vi "SAC-Configure Hardware (TDT).vi"(0 "Params":T1={"Fs (Hz)"=0.0, "atten (dB)"=0.0, "Waveform"=enum."Chirp", "Freq Res (Hz)"=0.0, "Order"=0, "Averages"=0, "seed"=-1, "Window"={"Type"=enum."None", "Length (ms)"=0.0, "Center (ms)"=0.0}, "Mic gain"=0.0, "Mic sens"=0.0}, 11 "error in (no error)":errorcluster) -> (4 "Stimulus":dbl[](array[numeric]), 6 "Sample Rate (Hz)":dbl, 8 "pts/rep":i32, 10 "reps/frame":i32, 15 "error out":errorcluster)   [LabVIEW 2020]
uses:
  Typedefs/SAC-Parameters.ctl
  HRTF VIs/Typedefs/HRTF-Waveform.ctl
  HRTF VIs/Typedefs/HRTF-Window.ctl
  HRTF VIs/Typedefs/HRTF-Window Type.ctl
  PXI DAQ VIs/TDT VIs/TDT-Signal Bank Action.ctl
  Typedefs/SAC-Hardware Config (TDT).ctl
  PXI DAQ VIs/TDT VIs/Typedefs/TDT-Output source.ctl
  PXI DAQ VIs/TDT VIs/Typedefs/TDT-Device ID.ctl
  PXI DAQ VIs/TDT VIs/Typedefs/TDT-Device Config.ctl
  PXI DAQ VIs/TDT VIs/Typedefs/TDT-Input source.ctl
  Utility VIs/Math VIs/dB to Linear (scalar).vi
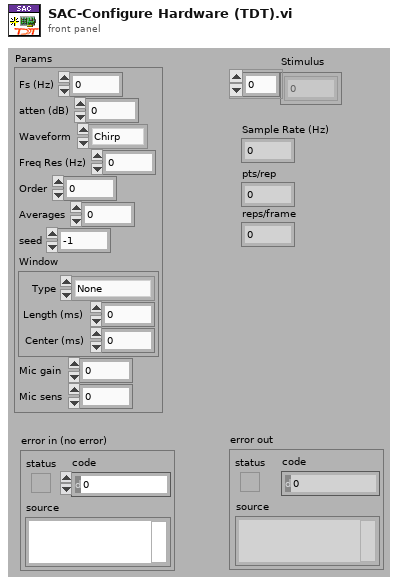
[diagram p1: front panel]
types:
  T1 = typedef "SAC-Parameters.ctl" = cluster{"Fs (Hz)":dbl, "atten (dB)":dbl, "Waveform":T2, "Freq Res (Hz)":dbl, "Order":i32, "Averages":i32, "seed":i64, "Window":T3, "Mic gain":dbl, "Mic sens":dbl}
  T2 = typedef "HRTF-Waveform.ctl" = enum16{"Chirp", "MLS"}
  T3 = typedef "HRTF-Window.ctl" = cluster{"Type":T4, "Length (ms)":dbl, "Center (ms)":dbl}
  T4 = typedef "HRTF-Window Type.ctl" = enum16{"None", "Rectangle", "Hanning"}
  T5 = typedef "TDT-Device Config.ctl" = cluster{"Output":T6, "Input":T8}
  T6 = typedef "TDT-Output source.ctl" = cluster{"Device":T7, "Num":i32}
  T7 = typedef "TDT-Device ID.ctl" = enum16{"None", "PA5", "RP2", "RL2", "RA16", "RV8", "RX5", "RX6", "RX7", "RX8", "RZ2", "RZ5", "RZ6"}
  T8 = typedef "TDT-Input source.ctl" = enum16{"Front Panel", "RA4LI", "RA16LI"}
  T9 = typedef "SAC-Hardware Config (TDT).ctl" = cluster{"Output":T6, "Speaker":cluster{"Channel":i32, "Primary mux":i32, "Secondary mux":i32}, "Cal mic":i32}
  T10 = typedef "TDT-Signal Bank Action.ctl" = enum16{"Init", "Write", "Read", "Rewrite", "Reset", "Recycle", "Ramp up", "Ramp down", "Zero"}
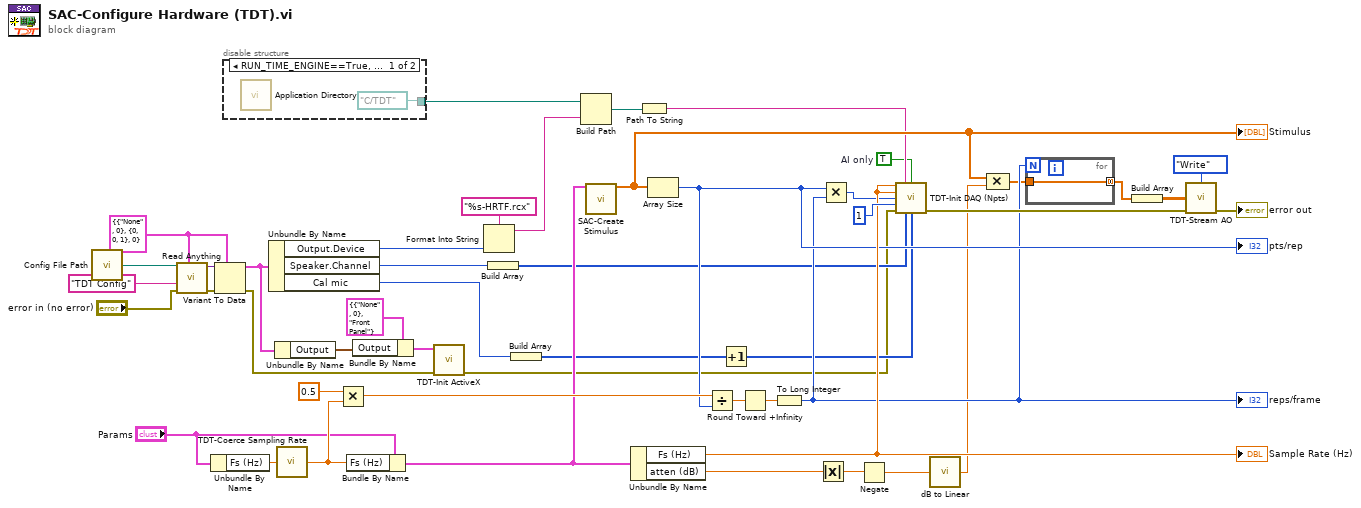
[diagram p0: block diagram]
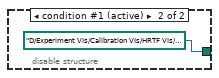
[diagram p2: hidden frame]
diagram:
  w8 = TRUE  # AI only
  w21 = T9 {"Output"={"Device"=enum."None", "Num"=0}, "Speaker"={"Channel"=0, "Primary mux"=0, "Secondary mux"=1}, "Cal mic"=0} ("TDT")
  n1 = call "Config File Path.vi"() -> ("Default config file name"=w25:path)  [unwired: 1 in]
  n2 = call "Read Anything.vi"("Type of Anything"=w21, "Error In"="error in (no error)", "Section Name (Name of \"Type of Anything\")"="TDT Config" ("Section Name (Name of \"Type of Anything\")"), "Path (dialog)"=w25) -> ("Error Out"=w28:errorcluster, "Anything"=w27:variant)  [unwired: 5 in, 1 out]
  n3 = Unbundle By Name("Params") -> ("Fs (Hz)"=w48:dbl)
  n4 = Variant To Data(error in=w28, type=w21, Variant=w27) -> (data=w3:T9, error out=w2:errorcluster)
  n5 = disable-structure shown="RUN_TIME_ENGINE==True, Default" {
    disable-tunnel: [path "C:/TDT" path "D:/Experiment VIs/Calibration VIs/HRTF VIs/rpfiles"] -> w18
    frame condition #0 {
      n6 = call <vilib>:"Application Directory.vi"() -> ()  [unwired: 1 out]
    }
    frame condition #1 (active) {
    }
  }
  n7 = Unbundle By Name(w3) -> ("Output.Device"=w15:T7, "Speaker.Channel"=w20:i32, "Cal mic"=w10:i32)
  n8 = Unbundle By Name(w3) -> ("Output"=w6:T6)
  n9 = call "TDT-Coerce Sampling Rate.vi"("Fs (Hz)"=w48) -> ("Coerced"=w38:dbl)
  n10 = Multiply(x=0.5, y=w38) -> (x*y=w36:dbl)
  n11 = Bundle By Name(cluster="Params", "Fs (Hz)"=w38) -> (w23:T1)
  n12 = Bundle By Name(cluster=T5 {"Output"={"Device"=enum."None", "Num"=0}, "Input"=enum."Front Panel"} ("TDT-Device Config"), "Output"=w6) -> (w5:T5)
  n13 = call "TDT-Init ActiveX.vi"("TDT-Device Config"=w5, "error in (no error)"=w2) -> ("error out"=w1:errorcluster)  [unwired: 10 in, 3 out]
  n14 = Format Into String(format string="%s-HRTF.rcx", w15) -> (resulting string=w14:string)  [unwired: 2 in, 1 out]
  n15 = Build Array(w20) -> (w19:i32[])
  n16 = Build Array(w10) -> (w9:i32[])
  n17 = Build Path(base path=w18, name or relative path=w14) -> (appended path=w13:path)
  n18 = call "SAC-Create Stimulus.vi"("Params"=w23) -> ("Stimulus"=w22:dbl[])  [unwired: 9 in, 5 out]
  "Stimulus" <- w22
  n19 = Unbundle By Name(w23) -> ("Fs (Hz)"=w46:dbl, "atten (dB)"=w45:dbl)
  "Sample Rate (Hz)" <- w46
  n20 = Path To String(path=w13) -> (string=w12:string)
  n21 = Array Size(array=w22) -> (size(s)=w32:i32)
  "pts/rep" <- w32
  n22 = Divide(x=w36, y=w32) -> (x/y=w35:dbl)
  n23 = Increment(x=w9) -> (x+1=w7:i32[])
  n24 = Round Toward +Infinity(x=w35) -> (ceil(x): smallest int >= x=w34:dbl)
  n25 = To Long Integer(number=w34) -> (32bit integer=w31:i32)
  "reps/frame" <- w31
  n26 = Absolute Value(x=w45) -> (abs(x)=w43:dbl)
  n27 = Multiply(x=w32, y=w31) -> (x*y=w33:i32)
  n28 = Negate(x=w43) -> (-x=w44:dbl)
  n29 = call "TDT-Init DAQ (Npts).vi"("AO Fs (Hz)"=w46, "Circuit"=w12, "AI only"=w8, "AI Fs (Hz)"=w46, "Num AO Pts"=w33, "Num AO Buffers"=1, "error in (no error)"=w1, "AO Channels"=w19, "AI Channels"=w7) -> ("error out"=w41:errorcluster)  [unwired: 2 in, 4 out]
  n30 = call-poly "dB to Linear.vi"("dB"=w44) -> ("linear"=w11:dbl)
  n31 = Compound Arithmetic op=MULTIPLY(w22, w11) -> (w30:dbl[])
  n32 = for {
    N: w31 -> [_]
    tunnel: w30 -> [w51]
    tunnel: [w51] -> w29 mode=concatenating
  }
  n33 = Build Array(w29) -> (w39:dbl[][])
  n34 = call "TDT-Stream AO.vi"("Action"=TDT-Signal_Bank_Action."Write", "Output array"=w39, "error in (no error)"=w41) -> ("error out"=→"error out":errorcluster)  [unwired: 12 in]
